vi "run iterator.vi"(8 "error in (no error)":errorcluster, 11 "SPARC4_GEI in":refnum<class "SPARC4_GEI.lvclass">) -> (0 "error out":errorcluster, 3 "SPARC4_GEI out":refnum<class "SPARC4_GEI.lvclass">)   [LabVIEW 2018, in "SPARC4_GEI.lvclass"]
uses:
  SPARC4_GEI.lvclass
  SPARC4_GEI.lvclass/SPARC4_GEI.ctl
  FWCS_ACS_Iterator/FWCS_ACS_Iterator.lvclass/FWCS_ACS_Iterator.ctl
  Filter_Wheel/Filter_Wheel.lvclass/Filter_Wheel.ctl
  Interface/Interface.lvclass/Interface.ctl
  FWCS_ACS_Iterator/FWCS_ACS_Iterator.lvclass
  Filter_Wheel/Filter_Wheel.lvclass
  Channel GUI/Channel GEI.lvclass
  RxTx/RxTx.lvclass
  Interface/Interface.lvclass
panel:
  in  "Filter":u16(ring) items=["U"=1, "B"=2, "V"=3, "R"=4, "I"=5, "Clear"=6]
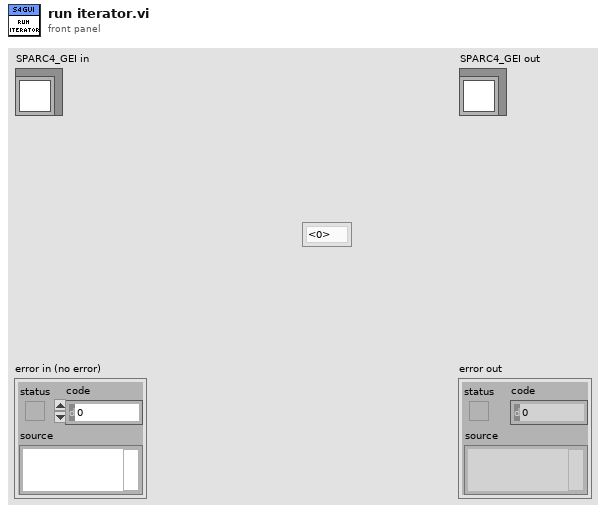
[diagram p1: front panel]
types:
  T1 = cluster{"Select":bool, "Exp Time":u16, "#Frames":u16, "Sufix":string, "Filter":u16}[]
  T2 = cluster{"Select":bool, "Exp Time":u16, "#Frames":u16, "Sufix":string, "Filter":u16}
  T3 = cluster{"COOLER_POWER_STATUS":u16, "TEMP":i32, "EXPTIME":dbl, "#FRAMES":u32, "#CUBES":u32}
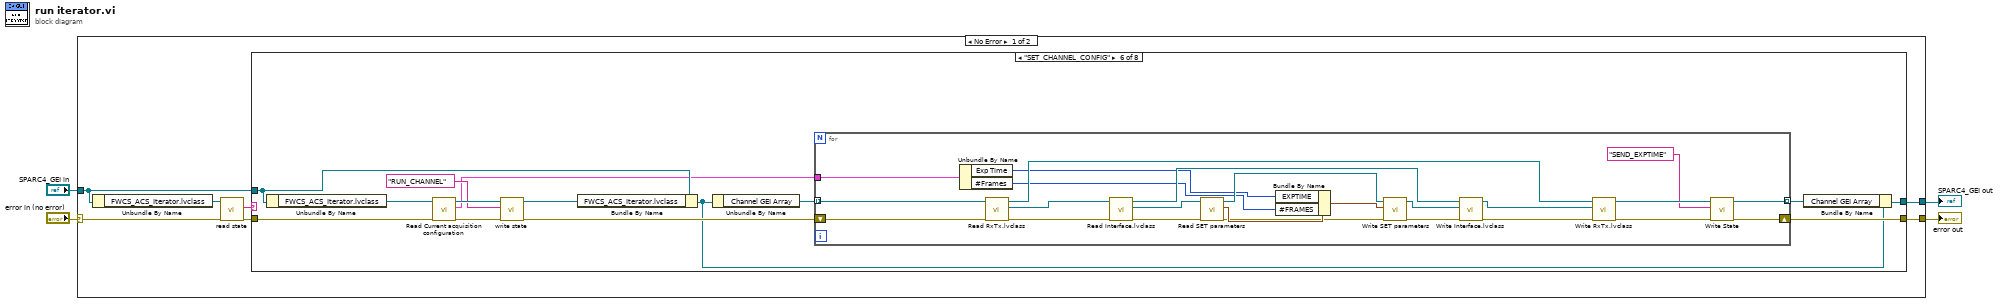
[diagram p0: block diagram]
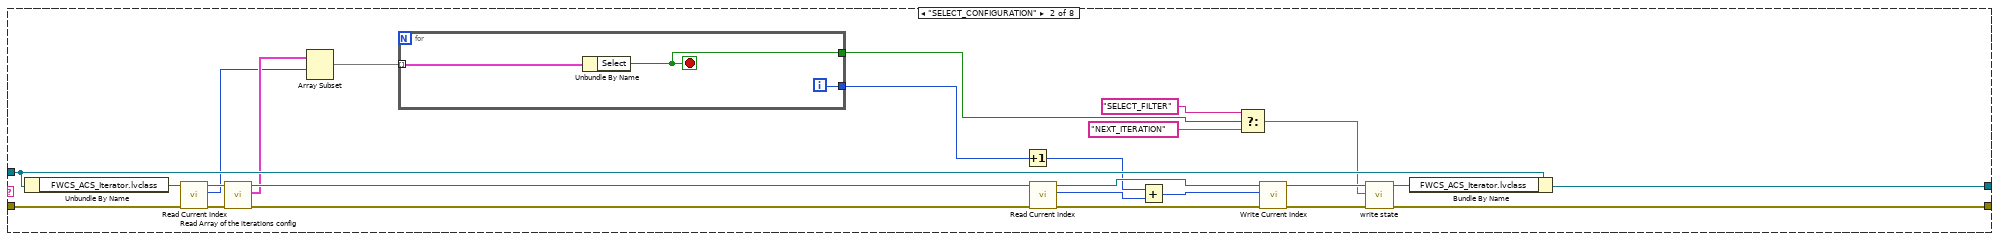
[diagram p3: hidden frame]
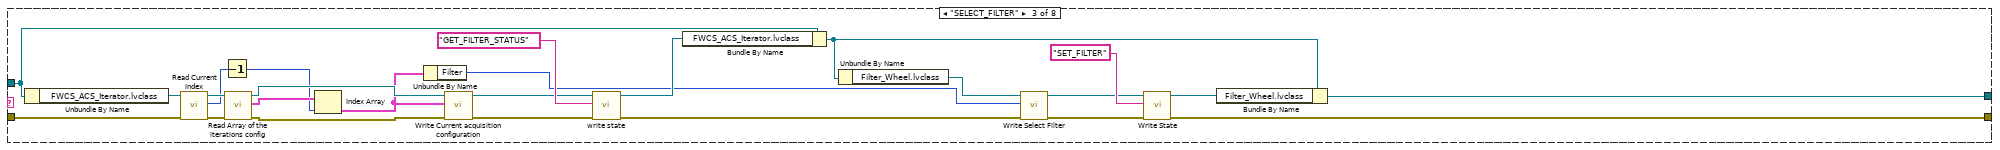
[diagram p4: hidden frame]
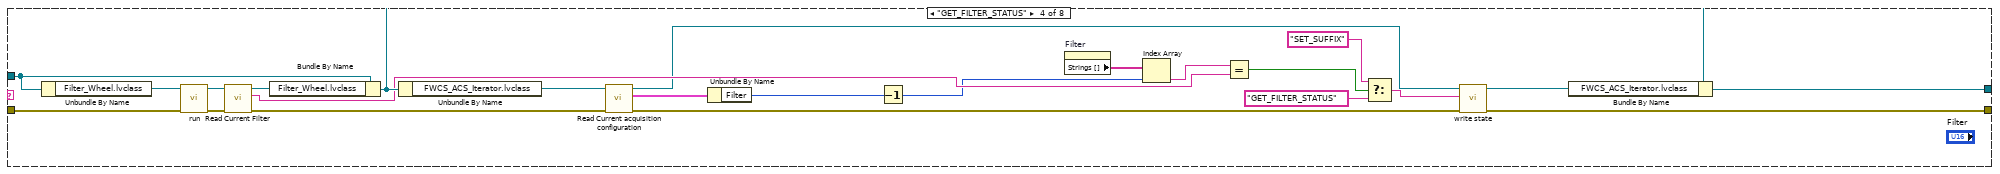
[diagram p5: hidden frame]
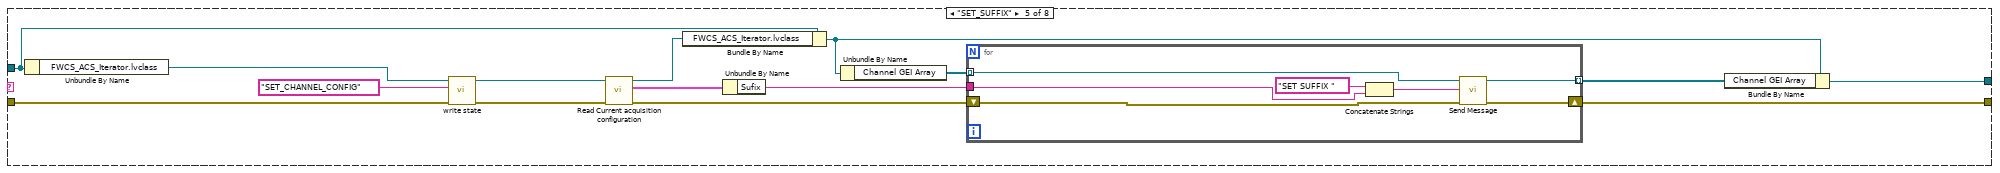
[diagram p6: hidden frame]
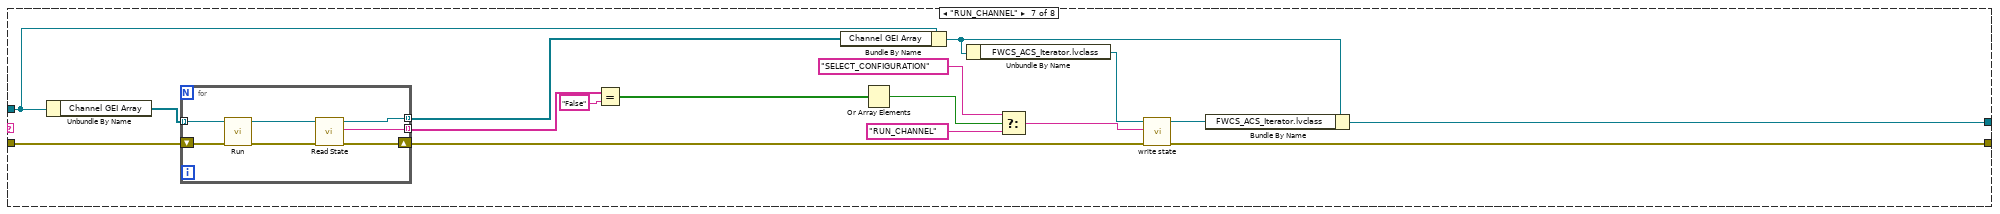
[diagram p7: hidden frame]
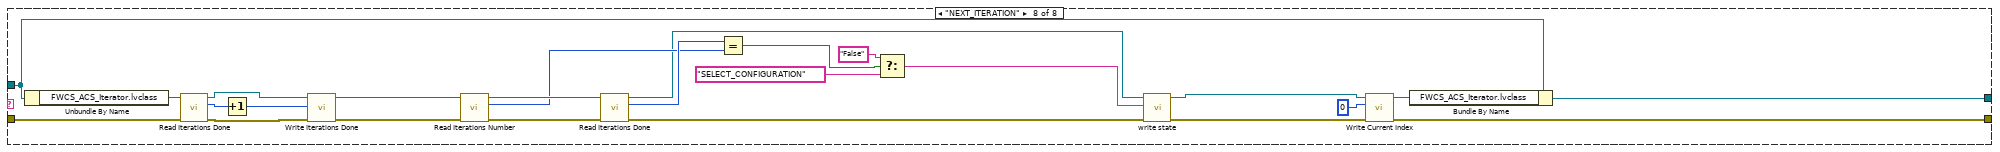
[diagram p8: hidden frame]
diagram:
  n1 = case shown="No Error" "error in (no error)" {
    selector: "error in (no error)" -> [w10 w201]
    tunnel: [w5 w201] -> w3
    tunnel: [w6 w200] -> w1
    tunnel: "SPARC4_GEI in" -> [w8 w200]
    frame No Error {
      n2 = Unbundle By Name(w8) -> ("FWCS_ACS_Iterator.lvclass"=w11:refnum<class "FWCS_ACS_Iterator.lvclass">)
      n3 = call "read state.vi"("error in (no error)"=w10, "FWCS_ACS_Iterator in"=w11) -> ("error out"=w7:errorcluster, "State"=w9:string)  [unwired: 7 in, 1 out]
      n4 = case shown="\"SET_CHANNEL_CONFIG\"" w9 {
        tunnel: w8 -> [w13 w36 w66 w86 w98 w116 w164 w198]
        tunnel: w7 -> [w12 w31 w60 w90 w101 w125 w167 w183]
        tunnel: [w13 w35 w47 w73 w92 w122 w151 w199] -> w6
        tunnel: [w12 w24 w46 w74 w91 w121 w152 w179] -> w5
        frame "False", Default {
        }
        frame "SELECT_CONFIGURATION" {
          n5 = Unbundle By Name(w36) -> ("FWCS_ACS_Iterator.lvclass"=w32:refnum<class "FWCS_ACS_Iterator.lvclass">)
          n6 = call "Read Current Index.vi"("error in (no error)"=w31, "FWCS_ACS_Iterator in"=w32) -> ("error out"=w34:errorcluster, "Current Index"=w26:u16, "FWCS_ACS_Iterator out"=w33:refnum<class "FWCS_ACS_Iterator.lvclass">)  [unwired: 7 in]
          n7 = call "Read Array of the iterations config.vi"("error in (no error)"=w34, "FWCS_ACS_Iterator in"=w33) -> ("error out"=w37:errorcluster, "Array of the iterations config"=w30:T1, "FWCS_ACS_Iterator out"=w38:refnum<class "FWCS_ACS_Iterator.lvclass">)  [unwired: 7 in]
          n8 = Array Subset(array=w30, index=w26) -> (w29:T1)  [unwired: 1 in]
          n9 = for {
            tunnel: w29 -> [w41] mode=indexing
            tunnel: [w40] -> w15
            tunnel: [w39] -> w19
            i -> [w40]
            stop <- w39 stop-if-true
            n10 = Unbundle By Name(w41) -> ("Select"=w39:bool)
          }
          n11 = Increment(x=w15) -> (x+1=w14:i32)
          n12 = call "Read Current Index.vi"("error in (no error)"=w37, "FWCS_ACS_Iterator in"=w38) -> ("error out"=w23:errorcluster, "Current Index"=w21:u16, "FWCS_ACS_Iterator out"=w22:refnum<class "FWCS_ACS_Iterator.lvclass">)  [unwired: 7 in]
          n13 = Add(x=w14, y=w21) -> (x+y=w25:i32)
          n14 = Select(t="SELECT_FILTER", s=w19, f="NEXT_ITERATION") -> (s? t:f=w16:string)
          n15 = call "Write Current Index.vi"("error in (no error)"=w23, "Current Index"=w25, "FWCS_ACS_Iterator in"=w22) -> ("error out"=w27:errorcluster, "FWCS_ACS_Iterator out"=w28:refnum<class "FWCS_ACS_Iterator.lvclass">)  [unwired: 7 in]
          n16 = call "write state.vi"("error in (no error)"=w27, "State"=w16, "FWCS_ACS_Iterator in"=w28) -> ("error out"=w24:errorcluster, "FWCS_ACS_Iterator out"=w20:refnum<class "FWCS_ACS_Iterator.lvclass">)  [unwired: 7 in]
          n17 = Bundle By Name(cluster=w36, "FWCS_ACS_Iterator.lvclass"=w20) -> (w35:refnum<class "SPARC4_GEI.lvclass">)
        }
        frame "SELECT_FILTER" {
          n18 = Unbundle By Name(w66) -> ("FWCS_ACS_Iterator.lvclass"=w61:refnum<class "FWCS_ACS_Iterator.lvclass">)
          n19 = call "Read Current Index.vi"("error in (no error)"=w60, "FWCS_ACS_Iterator in"=w61) -> ("error out"=w59:errorcluster, "Current Index"=w54:u16, "FWCS_ACS_Iterator out"=w58:refnum<class "FWCS_ACS_Iterator.lvclass">)  [unwired: 7 in]
          n20 = Decrement(x=w54) -> (x-1=w53:u16)
          n21 = call "Read Array of the iterations config.vi"("error in (no error)"=w59, "FWCS_ACS_Iterator in"=w58) -> ("error out"=w57:errorcluster, "Array of the iterations config"=w55:T1, "FWCS_ACS_Iterator out"=w56:refnum<class "FWCS_ACS_Iterator.lvclass">)  [unwired: 7 in]
          n22 = Index Array(array=w55, index=w53) -> (element=w43:T2)
          n23 = Unbundle By Name(w43) -> ("Filter"=w42:u16)
          n24 = call "Write Current acquisition configuration.vi"("error in (no error)"=w57, "Current acquisition configuration"=w43, "FWCS_ACS_Iterator in"=w56) -> ("error out"=w62:errorcluster, "FWCS_ACS_Iterator out"=w63:refnum<class "FWCS_ACS_Iterator.lvclass">)  [unwired: 7 in]
          n25 = call "write state.vi"("error in (no error)"=w62, "State"="GET_FILTER_STATUS", "FWCS_ACS_Iterator in"=w63) -> ("error out"=w44:errorcluster, "FWCS_ACS_Iterator out"=w64:refnum<class "FWCS_ACS_Iterator.lvclass">)  [unwired: 7 in]
          n26 = Bundle By Name(cluster=w66, "FWCS_ACS_Iterator.lvclass"=w64) -> (w49:refnum<class "SPARC4_GEI.lvclass">)
          n27 = Unbundle By Name(w49) -> ("Filter_Wheel.lvclass"=w50:refnum<class "Filter_Wheel.lvclass">)
          n28 = call "Write Select Filter.vi"("error in (no error)"=w44, "Select Filter"=w42, "Filter_Wheel in"=w50) -> ("error out"=w52:errorcluster, "Filter_Wheel out"=w45:refnum<class "Filter_Wheel.lvclass">)  [unwired: 7 in]
          n29 = call "Write State.vi"("error in (no error)"=w52, "State"="SET_FILTER", "Filter_Wheel in"=w45) -> ("error out"=w46:errorcluster, "Filter_Wheel out"=w48:refnum<class "Filter_Wheel.lvclass">)  [unwired: 7 in]
          n30 = Bundle By Name(cluster=w49, "Filter_Wheel.lvclass"=w48) -> (w47:refnum<class "SPARC4_GEI.lvclass">)
        }
        frame "GET_FILTER_STATUS" {
          n31 = Unbundle By Name(w86) -> ("Filter_Wheel.lvclass"=w89:refnum<class "Filter_Wheel.lvclass">)
          n32 = call "run.vi"("error in (no error)"=w90, "Filter_Wheel in"=w89) -> ("error out"=w88:errorcluster, "Filter_Wheel out"=w87:refnum<class "Filter_Wheel.lvclass">)  [unwired: 8 in]
          n33 = call "Read Current Filter.vi"("error in (no error)"=w88, "Filter_Wheel in"=w87) -> ("error out"=w82:errorcluster, "Current Filter"=w78:string, "Filter_Wheel out"=w85:refnum<class "Filter_Wheel.lvclass">)  [unwired: 7 in]
          n34 = Bundle By Name(cluster=w86, "Filter_Wheel.lvclass"=w85) -> (w84:refnum<class "SPARC4_GEI.lvclass">)
          n35 = Unbundle By Name(w84) -> ("FWCS_ACS_Iterator.lvclass"=w83:refnum<class "FWCS_ACS_Iterator.lvclass">)
          n36 = call "Read Current acquisition configuration.vi"("error in (no error)"=w82, "FWCS_ACS_Iterator in"=w83) -> ("error out"=w77:errorcluster, "Current acquisition configuration"=w81:T2, "FWCS_ACS_Iterator out"=w76:refnum<class "FWCS_ACS_Iterator.lvclass">)  [unwired: 7 in]
          n37 = Unbundle By Name(w81) -> ("Filter"=w68:u16)
          n38 = Decrement(x=w68) -> (x-1=w67:u16)
          n39 = property on="Filter" class="Ring (strict)"() -> ("Strings []"=w80:string[])  [unwired: 2 in, 2 out]
          n40 = Index Array(array=w80, index=w67) -> (element=w79:string)
          n41 = Equal?(x=w79, y=w78) -> (x = y?=w72:bool)
          n42 = Select(t="SET_SUFFIX", s=w72, f="GET_FILTER_STATUS") -> (s? t:f=w69:string)
          n43 = call "write state.vi"("error in (no error)"=w77, "State"=w69, "FWCS_ACS_Iterator in"=w76) -> ("error out"=w74:errorcluster, "FWCS_ACS_Iterator out"=w75:refnum<class "FWCS_ACS_Iterator.lvclass">)  [unwired: 7 in]
          n44 = Bundle By Name(cluster=w84, "FWCS_ACS_Iterator.lvclass"=w75) -> (w73:refnum<class "SPARC4_GEI.lvclass">)
        }
        frame "SET_SUFFIX" {
          n45 = Unbundle By Name(w98) -> ("FWCS_ACS_Iterator.lvclass"=w102:refnum<class "FWCS_ACS_Iterator.lvclass">)
          n46 = call "write state.vi"("error in (no error)"=w101, "State"="SET_CHANNEL_CONFIG", "FWCS_ACS_Iterator in"=w102) -> ("error out"=w99:errorcluster, "FWCS_ACS_Iterator out"=w100:refnum<class "FWCS_ACS_Iterator.lvclass">)  [unwired: 7 in]
          n47 = call "Read Current acquisition configuration.vi"("error in (no error)"=w99, "FWCS_ACS_Iterator in"=w100) -> ("error out"=w95:errorcluster, "Current acquisition configuration"=w105:T2, "FWCS_ACS_Iterator out"=w97:refnum<class "FWCS_ACS_Iterator.lvclass">)  [unwired: 7 in]
          n48 = Bundle By Name(cluster=w98, "FWCS_ACS_Iterator.lvclass"=w97) -> (w96:refnum<class "SPARC4_GEI.lvclass">)
          n49 = Unbundle By Name(w105) -> ("Sufix"=w93:string)
          n50 = Unbundle By Name(w96) -> ("Channel GEI Array"=w104:refnum<class "Channel GEI.lvclass">[])
          n51 = for {
            tunnel: w104 -> [w112] mode=indexing
            shift-right: [w110] -> w91
            shift-left: w95 -> [w111]
            tunnel: [w109] -> w103 mode=indexing
            tunnel: w93 -> [w107]
            n52 = Concatenate Strings("SET SUFFIX ", w107) -> (w106:string)
            n53 = call "Send Message.vi"("error in (no error)"=w111, "Message"=w106, "Channel GUI in"=w112) -> ("error out"=w110:errorcluster, "Channel GUI out"=w109:refnum<class "Channel GEI.lvclass">)  [unwired: 7 in]
          }
          n54 = Bundle By Name(cluster=w96, "Channel GEI Array"=w103) -> (w92:refnum<class "SPARC4_GEI.lvclass">)
        }
        frame "SET_CHANNEL_CONFIG" {
          n55 = Unbundle By Name(w116) -> ("FWCS_ACS_Iterator.lvclass"=w126:refnum<class "FWCS_ACS_Iterator.lvclass">)
          n56 = call "Read Current acquisition configuration.vi"("error in (no error)"=w125, "FWCS_ACS_Iterator in"=w126) -> ("error out"=w120:errorcluster, "Current acquisition configuration"=w113:T2, "FWCS_ACS_Iterator out"=w119:refnum<class "FWCS_ACS_Iterator.lvclass">)  [unwired: 7 in]
          n57 = call "write state.vi"("error in (no error)"=w120, "State"="RUN_CHANNEL", "FWCS_ACS_Iterator in"=w119) -> ("error out"=w118:errorcluster, "FWCS_ACS_Iterator out"=w114:refnum<class "FWCS_ACS_Iterator.lvclass">)  [unwired: 7 in]
          n58 = Bundle By Name(cluster=w116, "FWCS_ACS_Iterator.lvclass"=w114) -> (w115:refnum<class "SPARC4_GEI.lvclass">)
          n59 = Unbundle By Name(w115) -> ("Channel GEI Array"=w124:refnum<class "Channel GEI.lvclass">[])
          n60 = for {
            tunnel: w124 -> [w150] mode=indexing
            tunnel: [w132] -> w123 mode=indexing
            shift-right: [w133] -> w121
            shift-left: w118 -> [w149]
            tunnel: w113 -> [w129]
            n61 = Unbundle By Name(w129) -> ("Exp Time"=w128:u16, "#Frames"=w127:u16)
            n62 = call "Read RxTx.lvclass.vi"("error in (no error)"=w149, "Channel GUI in"=w150) -> ("error out"=w146:errorcluster, "RxTx.lvclass"=w147:refnum<class "RxTx.lvclass">, "Channel GUI out"=w148:refnum<class "Channel GEI.lvclass">)  [unwired: 7 in]
            n63 = call "Read Interface.lvclass.vi"("error in (no error)"=w146, "RxTx in"=w147) -> ("error out"=w141:errorcluster, "Interface.lvclass"=w142:refnum<class "Interface.lvclass">, "RxTx out"=w145:refnum<class "RxTx.lvclass">)  [unwired: 7 in]
            n64 = call "Read SET parameters.vi"("error in (no error)"=w141, "Interface in"=w142) -> ("error out"=w135:errorcluster, "SET parameters"=w137:T3, "Interface out"=w138:refnum<class "Interface.lvclass">)  [unwired: 7 in]
            n65 = Bundle By Name(cluster=w137, "EXPTIME"=w128, "#FRAMES"=w127) -> (w136:T3)
            n66 = call "Write SET parameters.vi"("error in (no error)"=w135, "SET parameters"=w136, "Interface in"=w138) -> ("error out"=w140:errorcluster, "Interface out"=w139:refnum<class "Interface.lvclass">)  [unwired: 7 in]
            n67 = call "Write Interface.lvclass.vi"("error in (no error)"=w140, "Interface.lvclass"=w139, "RxTx in"=w145) -> ("error out"=w144:errorcluster, "RxTx out"=w143:refnum<class "RxTx.lvclass">)  [unwired: 7 in]
            n68 = call "Write RxTx.lvclass.vi"("error in (no error)"=w144, "RxTx.lvclass"=w143, "Channel GUI in"=w148) -> ("error out"=w134:errorcluster, "Channel GUI out"=w131:refnum<class "Channel GEI.lvclass">)  [unwired: 7 in]
            n69 = call "Write State.vi"("error in (no error)"=w134, "State"="SEND_EXPTIME", "Channel GEI in"=w131) -> ("error out"=w133:errorcluster, "Channel GEI out"=w132:refnum<class "Channel GEI.lvclass">)  [unwired: 7 in]
          }
          n70 = Bundle By Name(cluster=w115, "Channel GEI Array"=w123) -> (w122:refnum<class "SPARC4_GEI.lvclass">)
        }
        frame "RUN_CHANNEL" {
          n71 = Unbundle By Name(w164) -> ("Channel GEI Array"=w166:refnum<class "Channel GEI.lvclass">[])
          n72 = for {
            tunnel: w166 -> [w173] mode=indexing
            tunnel: [w170] -> w165 mode=indexing
            shift-right: [w169] -> w153
            shift-left: w167 -> [w174]
            tunnel: [w168] -> w159 mode=indexing
            n73 = call "Run.vi"("error in (no error)"=w174, "Channel GUI in"=w173) -> ("error out"=w172:errorcluster, "Channel GUI out"=w171:refnum<class "Channel GEI.lvclass">)  [unwired: 8 in]
            n74 = call "Read State.vi"("error in (no error)"=w172, "Channel GEI in"=w171) -> ("error out"=w169:errorcluster, "State"=w168:string, "Channel GEI out"=w170:refnum<class "Channel GEI.lvclass">)  [unwired: 7 in]
          }
          n75 = Equal?(x=w159, y="False") -> (x = y?=w158:bool[])
          n76 = Bundle By Name(cluster=w164, "Channel GEI Array"=w165) -> (w163:refnum<class "SPARC4_GEI.lvclass">)
          n77 = Or Array Elements(Boolean array=w158) -> (logical OR=w157:bool)
          n78 = Unbundle By Name(w163) -> ("FWCS_ACS_Iterator.lvclass"=w162:refnum<class "FWCS_ACS_Iterator.lvclass">)
          n79 = Select(t="SELECT_CONFIGURATION", s=w157, f="RUN_CHANNEL") -> (s? t:f=w154:string)
          n80 = call "write state.vi"("error in (no error)"=w153, "State"=w154, "FWCS_ACS_Iterator in"=w162) -> ("error out"=w152:errorcluster, "FWCS_ACS_Iterator out"=w161:refnum<class "FWCS_ACS_Iterator.lvclass">)  [unwired: 7 in]
          n81 = Bundle By Name(cluster=w163, "FWCS_ACS_Iterator.lvclass"=w161) -> (w151:refnum<class "SPARC4_GEI.lvclass">)
        }
        frame "NEXT_ITERATION" {
          n82 = Unbundle By Name(w198) -> ("FWCS_ACS_Iterator.lvclass"=w184:refnum<class "FWCS_ACS_Iterator.lvclass">)
          n83 = call "Read Iterations Done.vi"("error in (no error)"=w183, "FWCS_ACS_Iterator in"=w184) -> ("error out"=w188:errorcluster, "Iterations Done"=w186:u16, "FWCS_ACS_Iterator out"=w187:refnum<class "FWCS_ACS_Iterator.lvclass">)  [unwired: 7 in]
          n84 = Increment(x=w186) -> (x+1=w185:u16)
          n85 = call "Write Iterations Done.vi"("error in (no error)"=w188, "Iterations Done"=w185, "FWCS_ACS_Iterator in"=w187) -> ("error out"=w181:errorcluster, "FWCS_ACS_Iterator out"=w182:refnum<class "FWCS_ACS_Iterator.lvclass">)  [unwired: 7 in]
          n86 = call "Read Iterations Number.vi"("error in (no error)"=w181, "FWCS_ACS_Iterator in"=w182) -> ("error out"=w197:errorcluster, "Iterations Number"=w194:u16, "FWCS_ACS_Iterator out"=w196:refnum<class "FWCS_ACS_Iterator.lvclass">)  [unwired: 7 in]
          n87 = call "Read Iterations Done.vi"("error in (no error)"=w197, "FWCS_ACS_Iterator in"=w196) -> ("error out"=w189:errorcluster, "Iterations Done"=w195:u16, "FWCS_ACS_Iterator out"=w190:refnum<class "FWCS_ACS_Iterator.lvclass">)  [unwired: 7 in]
          n88 = Equal?(x=w195, y=w194) -> (x = y?=w176:bool)
          n89 = Select(t="False", s=w176, f="SELECT_CONFIGURATION") -> (s? t:f=w191:string)
          n90 = call "write state.vi"("error in (no error)"=w189, "State"=w191, "FWCS_ACS_Iterator in"=w190) -> ("error out"=w180:errorcluster, "FWCS_ACS_Iterator out"=w177:refnum<class "FWCS_ACS_Iterator.lvclass">)  [unwired: 7 in]
          n91 = call "Write Current Index.vi"("error in (no error)"=w180, "Current Index"=u16 0, "FWCS_ACS_Iterator in"=w177) -> ("error out"=w179:errorcluster, "FWCS_ACS_Iterator out"=w178:refnum<class "FWCS_ACS_Iterator.lvclass">)  [unwired: 7 in]
          n92 = Bundle By Name(cluster=w198, "FWCS_ACS_Iterator.lvclass"=w178) -> (w199:refnum<class "SPARC4_GEI.lvclass">)
        }
      }
    }
    frame Error {
    }
  }
  "error out" <- w3
  "SPARC4_GEI out" <- w1
